vi "IsOddI64.vi"(4 "x":i64) -> (1 "Odd?":bool)   [LabVIEW 2017, in "GPComparison.lvlib"]
doc: "<B>Odd?</B> will be True if <B>x</B> is an odd integer.\n\nThis VI is inlined.\n\nSteen Schmidt\nGPower\n6/3 2013"
uses:
  GPComparison.lvlib
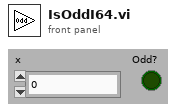
[diagram p1: front panel]
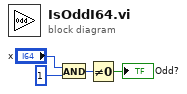
[diagram p0: block diagram]
diagram:
  n1 = And(x="x", y=i64 1) -> (x .and. y?=w4:i64)
  n2 = Not Equal To 0?(x=w4) -> (x != 0?=→"Odd?":bool)
